vi "Multiple Write in Loop.vi"() -> ()   [LabVIEW 2014, in "Arduino SoftwareSerial Wrapper.lvlib"]
uses:
  <vilib>/Aledyne-TSXperts/Arduino Compatible Compiler for LabVIEW/addons/Arduino SoftwareSerial Wrapper/Arduino SoftwareSerial Wrapper.lvlib
panel:
  out "Error Out":errorcluster
  in  "Error In":errorcluster
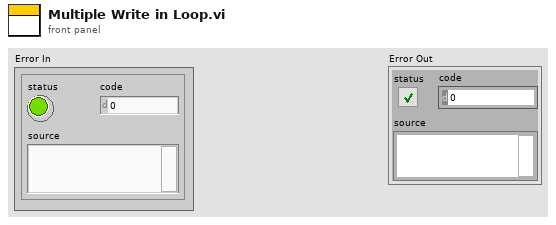
[diagram p1: front panel]
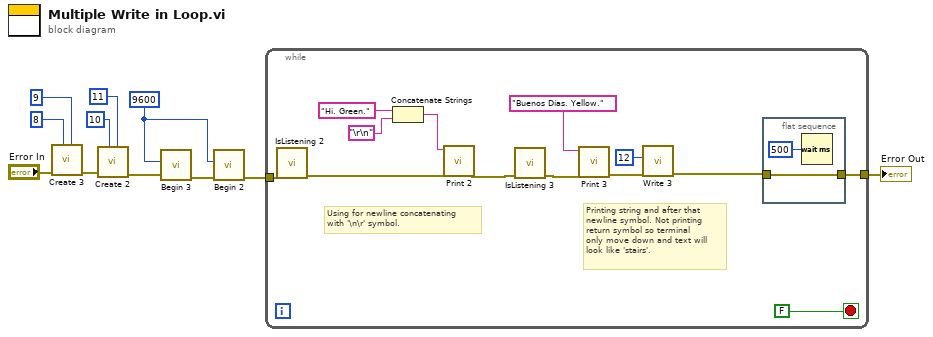
[diagram p0: block diagram]
diagram:
  w2 = u16 9600 ("Baudrate")
  n1 = call <vilib>:"Create 3.vi"("arduino TX pin"=u8 9, "arduino RX pin"=u8 8, "Error In"="Error In") -> ("Error Out"=w11:errorcluster)  [unwired: 8 in]
  n2 = call <vilib>:"Create 2.vi"("arduino TX pin"=u8 11, "arduino RX pin"=u8 10 ("arduino TX pin"), "Error In"=w11) -> ("Error Out"=w10:errorcluster)  [unwired: 8 in]
  n3 = call <vilib>:"Begin 3.vi"("Error In"=w10, "Baudrate"=w2) -> ("Error Out"=w9:errorcluster)  [unwired: 8 in]
  n4 = call <vilib>:"Begin 2.vi"("Error In"=w9, "Baudrate"=w2) -> ("Error Out"=w8:errorcluster)  [unwired: 8 in]
  n5 = while {
    tunnel: w8 -> [w24]
    tunnel: [w19] -> w1
    stop <- FALSE stop-if-true
    # "Using for newline concatenating\nwith '\\n\\r' symbol."
    # "Printing string and after that\nnewline symbol. Not printing\nreturn symbol so terminal\nonly move down and text will\nlook like 'stairs'."
    n6 = call <vilib>:"IsListening 2.vi"("Error In"=w24) -> ("Error Out"=w23:errorcluster)  [unwired: 9 in, 1 out]
    n7 = Concatenate Strings("Hi. Green." ("String to print"), "\r\n") -> (w15:string)
    n8 = call <vilib>:"Print 2.vi"("Error In"=w23, "String to print"=w15) -> ("Error Out"=w22:errorcluster)  [unwired: 9 in]
    n9 = call <vilib>:"IsListening 3.vi"("Error In"=w22) -> ("Error Out"=w21:errorcluster)  [unwired: 9 in, 1 out]
    n10 = call <vilib>:"Print 3.vi"("Error In"=w21, "String to print"="Buenos Días. Yellow.") -> ("Error Out"=w14:errorcluster)  [unwired: 9 in]
    n11 = call <vilib>:"Write 3.vi"("Error In"=w14, "Char to write"=u8 12) -> ("Error Out"=w13:errorcluster)  [unwired: 9 in]
    n12 = flat-sequence {
      tunnel: [w26] -> w19
      tunnel: w13 -> [w26]
      frame #0 {
        n13 = Wait (ms)(milliseconds to wait=u32 500) -> ()  [unwired: 1 out]
      }
    }
  }
  "Error Out" <- w1
